vi "Test Get Parallel Tests Enabeld Cretes if not Found.vi"(8 "error in (no error)":errorcluster, 11 "Configuration Manager Test in":refnum<class "Configuration Manager Test.lvclass">) -> (0 "error out":errorcluster, 3 "Configuration Manager Test out":refnum<class "Configuration Manager Test.lvclass">)   [LabVIEW 2020, in "Configuration Manager Test.lvclass"]
uses:
  Configuration Manager Test.lvclass
  C:/Program Files (x86)/National Instruments/LabVIEW 2020/vi.lib/Astemes/LUnit/Test Case.lvclass
  <vilib>/Astemes/LUnit/Test Case.lvclass/Test Case.ctl
  7bdc5723-55b7-4bdc-95a2-3da71d0506ac.vi
  <vilib>/Astemes/LUnit/Palette/Fail.vi
  <vilib>/Astemes/LUnit/Palette/Pass.vi
  <vilib>/Astemes/LUnit/Compare Variants.vi
  <vilib>/Astemes/LUnit/Describe Comparison.vi
  <vilib>/Astemes/LUnit/Set Assertion Type.vi
  <vilib>/Astemes/LUnit/Add test result.vi
  <vilib>/Astemes/LUnit/Variant to string.vi
  <vilib>/Astemes/LUnit/LUnit Record Assertion Result.vi
  <vilib>/Astemes/LUnit/LUnit Aggregate Assertion Results.vi
  <vilib>/Astemes/LUnit/Method Result/LUnit Merge Status.vi
  <vilib>/Astemes/LUnit/LUnit Concatenate result strings.vi
  <vilib>/Utility/Data Type/Get Type Information.vi
  <vilib>/Utility/LVClass/Get LV Class Name.vi
  source/User Interface/Configuration Manager/Configuration Manager.lvclass
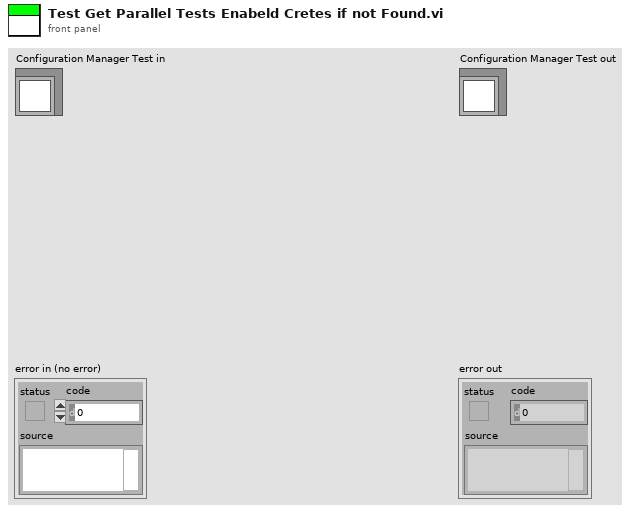
[diagram p1: front panel]
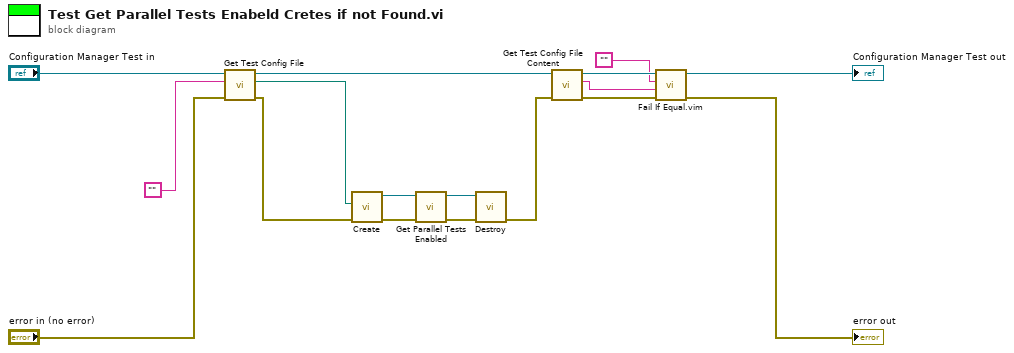
[diagram p0: block diagram]
diagram:
  n1 = call "Get Test Config File.vi"("error in (no error)"="error in (no error)", "File Content"="", "Configuration Manager Test in"="Configuration Manager Test in") -> ("error out"=w10:errorcluster, "File Path"=w6:path, "Configuration Manager Test out"=w4:refnum<class "Configuration Manager Test.lvclass">)  [unwired: 6 in]
  n2 = call "Create.vi"("error in (no error)"=w10, "configuration file path"=w6) -> ("error out"=w13:errorcluster, "Configuration Manager out"=w14:refnum<class "Configuration Manager.lvclass">)  [unwired: 8 in]
  n3 = call "Get Parallel Tests Enabled.vi"("error in (no error)"=w13, "Configuration Manager In"=w14) -> ("error out"=w11:errorcluster, "Configuration Manager Out"=w12:refnum<class "Configuration Manager.lvclass">)  [unwired: 7 in, 1 out]
  n4 = call "Destroy.vi"("error in (no error)"=w11, "Configuration Manager In"=w12) -> ("error out"=w9:errorcluster)  [unwired: 9 in]
  n5 = call "Get Test Config File Content.vi"("error in (no error)"=w9, "Configuration Manager Test in"=w4) -> ("error out"=w5:errorcluster, "File Content"=w1:string, "Configuration Manager Test out"=w3:refnum<class "Configuration Manager Test.lvclass">)  [unwired: 7 in]
  n6 = call "Fail If Equal.vim"("error in (no error)"=w5, "Actual"=w1, "Expected"="" ("File Content"), "LUnit Test Case In"=w3) -> ("error out"=→"error out":errorcluster, "LUnit Test Case Out"=→"Configuration Manager Test out":refnum<class "Configuration Manager Test.lvclass">)  [unwired: 6 in]
